vi "Memory.Pointer.Parameter Check.Offset.vi"(7 "calling vi name":string, 8 "error in (no error)":errorcluster, 10 "offset":u64 format="%d bytes", 11 "Pointer in":refnum<class "Memory.Pointer.lvclass">) -> (0 "error out":errorcluster, 2 "offset out":u64 format="%d bytes", 3 "Pointer out":refnum<class "Memory.Pointer.lvclass">)   [LabVIEW 2016, in "LabVIEW Memory Manager.lvlib" / "Memory.Pointer.lvclass"]
uses:
  Memory.Pointer.lvclass
  Memory.Pointer.lvclass/Memory.Pointer.ctl
  Typedefs/Memory.Pointer.Parameters.ctl
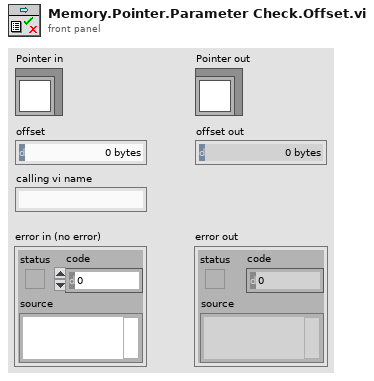
[diagram p1: front panel]
types:
  T1 = typedef "LabVIEW Memory Manager.lvlib/Memory.Pointer.lvclass/Memory.Pointer.Parameters.ctl" = enum16{"offset", "length", "size", "subset"}
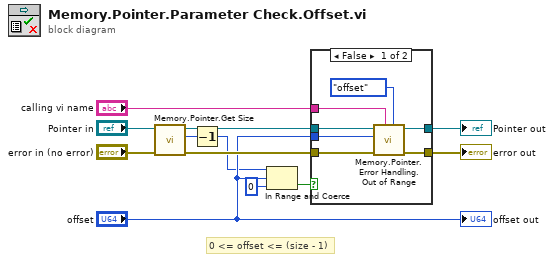
[diagram p0: block diagram]
diagram:
  # "0 <= offset <= (size - 1)"
  n1 = call "Memory.Pointer.Get Size.vi"("error in (no error)"="error in (no error)", "Pointer in"="Pointer in") -> ("error out"=w9:errorcluster, "size"=w8:u64, "Pointer out"=w12:refnum<class "Memory.Pointer.lvclass">)  [unwired: 7 in]
  n2 = Decrement(x=w8) -> (x-1=w1:u64)
  n3 = In Range and Coerce(upper limit=w1, x="offset", lower limit=u64 0) -> (In Range?=w11:bool)  [unwired: 1 out]
  n4 = case shown="False" w11 {
    tunnel: [w19 w21] -> w4
    tunnel: "calling vi name" -> [w18 _]
    tunnel: w9 -> [w17 w21]
    tunnel: "offset" -> [w15 _]
    tunnel: w12 -> [w14 w20]
    tunnel: [w13 w20] -> w3
    frame False {
      n5 = call "Memory.Pointer.Error Handling.Out of Range.vi"("parameter"=Memory.Pointer.Parameters."offset", "source vi name"=w18, "error in (no error)"=w17, "value"=w15, "Pointer in"=w14) -> ("error out"=w19:errorcluster, "Pointer out"=w13:refnum<class "Memory.Pointer.lvclass">)  [unwired: 5 in]
    }
    frame True {
    }
  }
  "error out" <- w4
  "Pointer out" <- w3
  "offset out" <- "offset"
